vi "RT_IBN.vi"() -> ()   [LabVIEW 2016]
uses:
  <extravilib>/ChannelInstances/Stream-bool.lvlib
  HostRTCommunication/Commands.ctl
  HostRTCommunication/Command and Parameters.ctl
panel:
  out "error IO":errorcluster
  in  "AGC Enable":bool
  in  "Center Frequency":u32=101000000
  in  "Number of Averages":u32=4 min=1 max=255
  in  "Tuner AGC":bool
  in  "stop":bool
  out "Waveform Graph":dbl[](graph)
  out "Intensity Graph":dbl[][](graph)
  in  "Vertical Pointer Slide":dbl(slide) min=-99.0 max=1.0
  out "max value":dbl
  out "x+y":dbl format="%#_10p"
  out "min value":dbl
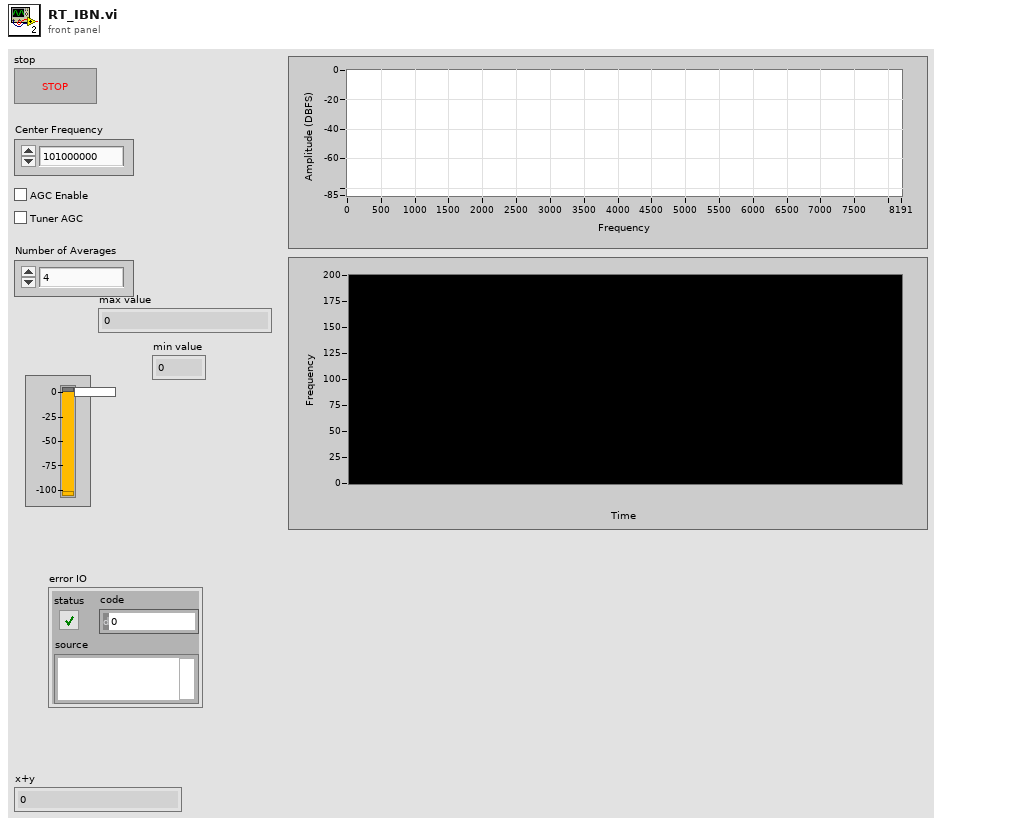
[diagram p1: front panel]
types:
  T1 = typedef "Stream-bool.lvlib/)Channel.ctl" = refnum<queue>
  T2 = typedef "Commands.ctl" = enum16{"Set Center Frequency", "Set AGC State", "Set Number Of Averages", "Set Tuner Gain Mode", "Set Frequency Correction", "Set Sample Rate", "Set Manual Gain Value"}
  T3 = typedef "Command and Parameters.ctl" = cluster{"Command":T2, "Command Parameters":variant[]}
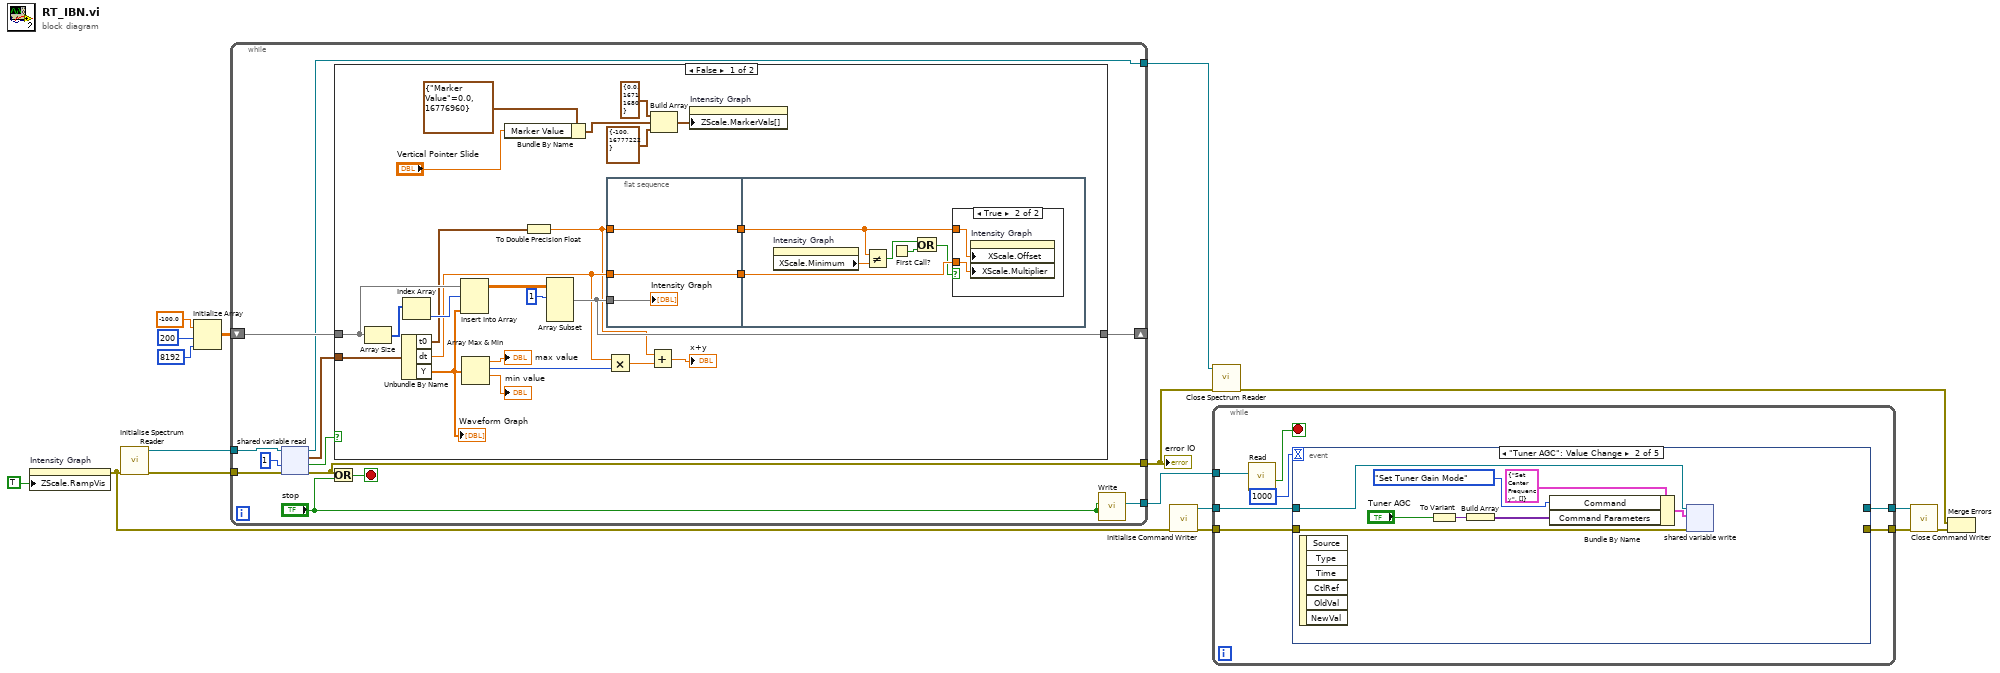
[diagram p0: block diagram]
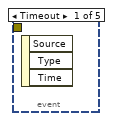
[diagram p2: hidden frame]
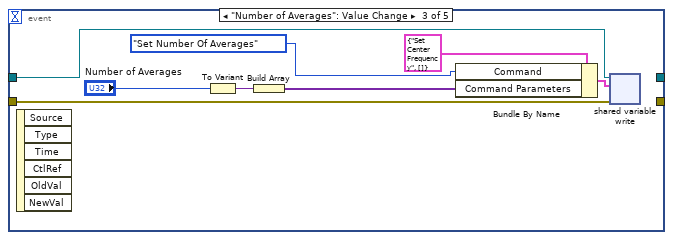
[diagram p3: hidden frame]
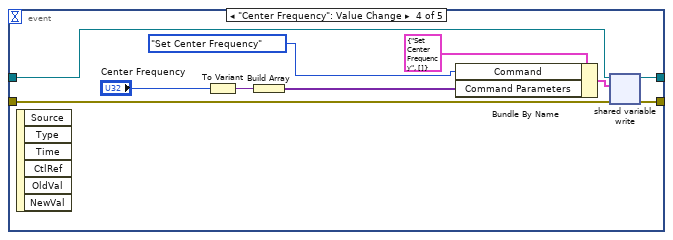
[diagram p4: hidden frame]
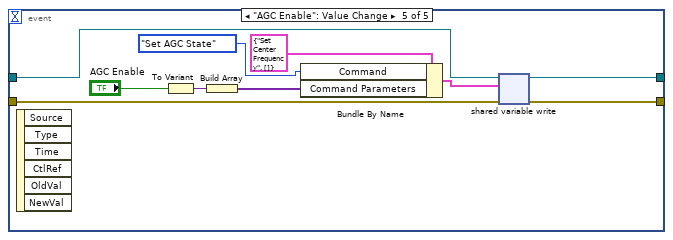
[diagram p5: hidden frame]
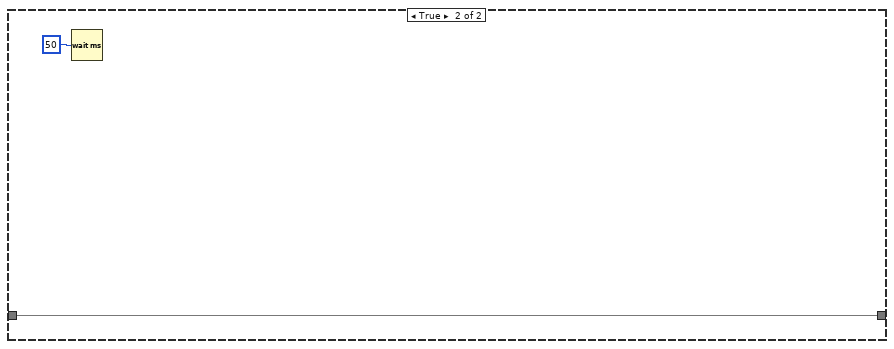
[diagram p7: hidden frame]
diagram:
  n1 = property on="Intensity Graph" class="IntGraph (strict)"("ZScale.RampVis"=TRUE ("Z Scale.Ramp Visible")) -> (error out=w2:errorcluster)  [unwired: 2 in, 1 out]
  n2 = call "Initialise Spectrum Reader.vi"("error in (no error)"=w2) -> ("error out"=w16:errorcluster, "Spectrum Reader"=w17:refnum<k21>)  [unwired: 9 in]
  n3 = Initialize Array(-100.0, 200 ("dimension size"), 8192 ("dimension size")) -> (w14:dbl[][])
  n4 = while {
    tunnel: w17 -> [w29]
    tunnel: w16 -> [w28]
    tunnel: [w22] -> w15
    tunnel: [w19] -> w1
    shift-right: [w25] -> _
    shift-left: w14 -> [w24]
    tunnel: [w21] -> w10
    stop <- w23 stop-if-true
    n5 = shared-variable-read(w29, w28, 1 ("timeout ms (-1)")) -> (w19:refnum<k21>, w22:errorcluster, w20:bool, w26:waveform(dbl))
    n6 = Or(x=w22, y="stop") -> (x .or. y?=w23:bool)
    n7 = case shown="False" w20 {
      tunnel: w26 -> [w34 _]
      tunnel: [w48 w66] -> w25
      tunnel: w24 -> [w53 w66]
      frame False {
        n8 = Array Size(array=w53) -> (size(s)=w52:i32[])
        n9 = Unbundle By Name(w34) -> ("t0"=w31:timestamp, "dt"=w32:dbl, "Y"=w33:dbl[])
        "Waveform Graph" <- w33
        n10 = Index Array(array=w52) -> (element=w51:i32)  [unwired: 1 in]
        n11 = Insert Into Array(array=w53, index (row)=w51, new element=w33) -> (w50:dbl[][])  [unwired: 1 in]
        n12 = Array Max & Min(array=w33) -> (max value=→"max value":dbl, max index (indices)=w38:i32, min value=→"min value":dbl)  [unwired: 1 out]
        n13 = Bundle By Name(cluster=cluster{"Marker Value":dbl, u32} {"Marker Value"=0.0, 16776960}, "Marker Value"="Vertical Pointer Slide") -> (w41:cluster{"Marker Value":dbl, u32})
        n14 = To Double Precision Float(number=w31) -> (double precision float=w30:dbl)
        n15 = Array Subset(array=w50, index (row)=1 ("index")) -> (w48:dbl[][])  [unwired: 3 in]
        n16 = flat-sequence {
          tunnel: [w56] -> w47
          tunnel: [w55] -> w46
          tunnel: w30 -> [w56]
          tunnel: w32 -> [w55]
          tunnel: w48 -> [w54]
          tunnel: w46 -> [w60]
          tunnel: w47 -> [w61]
          frame #0 {
            "Intensity Graph" <- w54
          }
          frame #1 {
            n17 = property on="Intensity Graph" class="IntGraph (strict)"() -> ("XScale.Minimum"=w62:dbl)  [unwired: 2 in, 2 out]
            n18 = Not Equal?(x=w61, y=w62) -> (x != y?=w58:bool)
            n19 = First Call?() -> (First Call?: T/F=w59:bool)
            n20 = Or(x=w58, y=w59) -> (x .or. y?=w57:bool)
            n21 = case shown="True" w57 {
              tunnel: w61 -> [_ w64]
              tunnel: w60 -> [_ w63]
              frame False {
              }
              frame True {
                n22 = property on="Intensity Graph" class="IntGraph (strict)"("XScale.Offset"=w64, "XScale.Multiplier"=w63) -> ()  [unwired: 2 in, 2 out]
              }
            }
          }
        }
        n23 = Multiply(x=w32, y=w38) -> (x*y=w37:dbl)
        n24 = Add(x=w30, y=w37) -> (x+y=→"x+y":dbl)
        n25 = Build Array(cluster{dbl, u32} {0.0, 16711680}, w41, cluster{i32, u32} {-100, 16777222}) -> (w43:cluster{"Marker Value":dbl, u32}[])
        n26 = property on="Intensity Graph" class="IntGraph (strict)"("ZScale.MarkerVals[]"=w43) -> ()  [unwired: 2 in, 2 out]
      }
      frame True {
        n27 = Wait (ms)(milliseconds to wait=u32 50) -> ()  [unwired: 1 out]
      }
    }
    n28 = call <extravilib>:"Write.vi"("last element? (F)"="stop", "element"="stop") -> ("channel"=w21:T1)  [unwired: 7 in, 2 out]
  }
  "error IO" <- w15
  n29 = call "Initialise Command Writer.vi"("error in (no error)"=w2) -> ("error out"=w9:errorcluster, "Refnum out"=w8:refnum<k21>)  [unwired: 9 in]
  n30 = call "Close Spectrum Reader.vi"("error in (no error)"=w15, "endpoint in"=w1) -> ("error out"=w5:errorcluster)  [unwired: 9 in]
  n31 = while {
    tunnel: w10 -> [w73]
    tunnel: w9 -> [w71]
    tunnel: w8 -> [w70]
    tunnel: [w69] -> w7
    tunnel: [w68] -> w6
    stop <- w67 stop-if-true
    n32 = call <extravilib>:"Read.vi"("channel"=w73) -> ("last element?"=w67:bool)  [unwired: 6 in, 4 out]
    n33 = event shown="[1] \"Tuner AGC\": Value Change" {
      selector: _ -> [_ _ _ _ _]
      dyn-events: _ -> [_ _ _ _ _]
      timeout: 1000 -> [_ _ _ _ _]
      tunnel: w71 -> [_ w75 w84 w99 w104]
      tunnel: w70 -> [_ w76 w83 w98 w105]
      tunnel: [_ _ _ w95 w102] -> w69
      tunnel: [_ _ _ w94 w103] -> w68
      event Timeout {
        n34 = event-data() -> ()  [unwired: 1 in, 3 out]
      }
      event "Tuner AGC": Value Change {
        n35 = event-data() -> ()  [unwired: 1 in, 6 out]
        n36 = To Variant(anything="Tuner AGC") -> (Variant=w79:variant)
        n37 = Build Array(w79) -> (w78:variant[])
        n38 = Bundle By Name(cluster=T3 {"Command"=enum."Set Center Frequency", "Command Parameters"=[]} ("Cluster"), "Command"=Commands."Set Tuner Gain Mode", "Command Parameters"=w78) -> (w80:T3)
        n39 = shared-variable-write(w76, w75, w80) -> ()  [unwired: 1 in, 3 out]
      }
      event "Number of Averages": Value Change {
        n40 = event-data() -> ()  [unwired: 1 in, 6 out]
        n41 = To Variant(anything="Number of Averages") -> (Variant=w87:variant)
        n42 = Build Array(w87) -> (w86:variant[])
        n43 = Bundle By Name(cluster=T3 {"Command"=enum."Set Center Frequency", "Command Parameters"=[]} ("Cluster"), "Command"=Commands."Set Number Of Averages", "Command Parameters"=w86) -> (w88:T3)
        n44 = shared-variable-write(w83, w84, w88) -> ()  [unwired: 1 in, 3 out]
      }
      event "Center Frequency": Value Change {
        n45 = event-data() -> ()  [unwired: 1 in, 6 out]
        n46 = To Variant(anything="Center Frequency") -> (Variant=w91:variant)
        n47 = Build Array(w91) -> (w90:variant[])
        n48 = Bundle By Name(cluster=T3 {"Command"=enum."Set Center Frequency", "Command Parameters"=[]} ("Cluster"), "Command"=Commands."Set Center Frequency", "Command Parameters"=w90) -> (w93:T3)
        n49 = shared-variable-write(w98, w99, w93) -> (w94:refnum<k21>, w95:errorcluster)  [unwired: 1 in, 1 out]
      }
      event "AGC Enable": Value Change {
        n50 = event-data() -> ()  [unwired: 1 in, 6 out]
        n51 = To Variant(anything="AGC Enable") -> (Variant=w107:variant)
        n52 = Build Array(w107) -> (w106:variant[])
        n53 = Bundle By Name(cluster=T3 {"Command"=enum."Set Center Frequency", "Command Parameters"=[]} ("Cluster"), "Command"=Commands."Set AGC State", "Command Parameters"=w106) -> (w108:T3)
        n54 = shared-variable-write(w105, w104, w108) -> (w103:refnum<k21>, w102:errorcluster)  [unwired: 1 in, 1 out]
      }
    }
  }
  n55 = call "Close Command Writer.vi"("error in (no error)"=w7, "Refnum in"=w6) -> ("error out"=w4:errorcluster)  [unwired: 9 in]
  n56 = Merge Errors(w5, w4) -> ()  [unwired: 1 out]
